vi "ResonanceAnalyzer.vi"() -> ()   [LabVIEW 2014]
uses:
  <vilib>/imath/engines/lvmath2/RunTimeEngine/Managers/WorkSpace/UID Generator.vi
  <vilib>/imath/engines/lvmath2/RunTimeEngine/RangeToken/NIMS_Range.vi
  <instcachedir>/0/NIMS_Range_9BCE657718DF4976A877346C61F22738.lvgen/NIMS_Range_9BCE657718DF4976A877346C61F22738_000.vi
  <vilib>/imath/engines/lvmath2/RunTimeEngine/RunTimeType/NIMS_RunTimeType_From StrictType (excl LVString).vi
  <instcachedir>/0/NIMS_RunTimeType_From StrictType (excl LVString)_15A5391EEA9C4AACB9955AC755B83D29.lvgen/NIMS_RunTimeType_From StrictType (excl LVString)_15A5391EEA9C4AACB9955AC755B83D29_000.vi
  <vilib>/imathl/engines/lvmath/Functions/Error Handling/Create Error.vi
  <vilib>/imath/engines/lvmath2/RunTimeEngine/LocalVariableDefStatement/MC_LocalVariableDefStatement_Display.vi
  <vilib>/imath/engines/lvmath2/RunTimeEngine/ArithmeticOperatorToken/NIMS_ArithmeticOperator_minus.vi
  <instcachedir>/0/NIMS_ArithmeticOperator_minus_39C0593E74DA4138ACA2AB742906488D.lvgen/NIMS_ArithmeticOperator_minus_39C0593E74DA4138ACA2AB742906488D_003.vi
  <vilib>/imath/engines/lvmath2/RunTimeEngine/BuiltInFunctions/randnormal/NIMS_randnormal(1,I32).vi
  <vilib>/imath/engines/lvmath2/RunTimeEngine/ErrorHandling/NIMS_Error From Error Code.vi
  <vilib>/imath/engines/lvmath2/RunTimeEngine/ArithmeticOperatorToken/NIMS_ArithmeticOperator_power(S).vi
  <instcachedir>/0/NIMS_ArithmeticOperator_power(S)_CAFE680B12A64A3A8F5E28A20C679B7D.lvgen/NIMS_ArithmeticOperator_power(S)_CAFE680B12A64A3A8F5E28A20C679B7D_014.vi
  <vilib>/imath/engines/lvmath2/RunTimeEngine/ArithmeticOperatorToken/NIMS_ArithmeticOperator_plus.vi
  <instcachedir>/0/NIMS_ArithmeticOperator_plus_48D6EAACA5D645B09F7EC9C016C2DEA8.lvgen/NIMS_ArithmeticOperator_plus_48D6EAACA5D645B09F7EC9C016C2DEA8_000.vi
  <vilib>/imath/engines/lvmath2/RunTimeEngine/ErrorHandling/NIMS_Create Error From Enums.vi
  <vilib>/imath/engines/lvmath2/RunTimeEngine/Managers/SymbolTable/Clear UID.vi
  <vilib>/imath/engines/lvmath2/RunTimeEngine/NodeEndStatement/NIMS_NodeEndStatement_Output.vi
  <instcachedir>/0/NIMS_NodeEndStatement_Output_53EC0D466D134D7ABD903AC30B43404B.lvgen/NIMS_NodeEndStatement_Output_53EC0D466D134D7ABD903AC30B43404B_000.vi
  <instcachedir>/0/NIMS_NodeEndStatement_Output_53EC0D466D134D7ABD903AC30B43404B.lvgen/NIMS_NodeEndStatement_Output_53EC0D466D134D7ABD903AC30B43404B_005.vi
  <vilib>/imath/engines/lvmath2/RunTimeEngine/ErrorHandling/NIMS_Finalize Error.vi
  <vilib>/Utility/file.llb/Read From Spreadsheet File (DBL).vi
  <vilib>/imath/engines/lvmath2/RunTimeEngine/Managers/SymbolTable/NIMS_WorkSpace.lvlib
panel:
  out "output cluster":cluster{"all rows":dbl[], "Array":dbl[]}={"all rows"=[425.0, 430.0, 435.0, 440.0, 445.0, 450.0, 455.0, 460.0, 465.0, 470.0, 475.0, 480.0, 485.0, 490.0, 495.0, 500.0, 505.0, 510.0, 515.0, 520.0, 525.0, 530.0, 535.0, 540.0, 545.0, 550.0, 555.0, 560.0, 565.0], "Array"=[0.00029010896046823345, 0.000307774576785936, 0.00032832543217633636, 0.0003525272075386067, 0.0003814382755160812, 0.000416561323783634, 0.0004600972655461633, 0.0005153884048945562, 0.0005877272439052437, 0.0006858979557065526, 0.0008251875476773748, 0.0010328740074356068, 0.0013523841688152917, 0.0017892153610694526, 0.0020107857493675313, 0.0016828151148900047, 0.0012753396459793623, 0.0009947134075484914, 0.0008111662113022912, 0.0006861595529584501, 0.0005967970519750586, 0.0005301782426142894, 0.0004787804413681282, 0.00043800311684869474, 0.0004049022123545997, 0.00037751685257886314, 0.00035449514124371066, 0.000334876933310768, 0.0003179625943458466]}
  out "XY Graph":cluster{dbl[], dbl[]}[](graph)=[{[425.0, 430.0, 435.0, 440.0, 445.0, 450.0, 455.0, 460.0, 465.0, 470.0, 475.0, 480.0, 485.0, 490.0, 495.0, 500.0, 505.0, 510.0, 515.0, 520.0, 525.0, 530.0, 535.0, 540.0, 545.0, 550.0, 555.0, 560.0, 565.0], [0.00032, 0.00034, 0.00034, 0.00036, 0.0004, 0.0004, 0.00046, 0.0005, 0.00059, 0.00066, 0.00082, 0.00102, 0.00141, 0.00177, 0.00199, 0.00173, 0.00124, 0.00103, 0.00079, 0.00067, 0.00061, 0.00051, 0.00046, 0.00039, 0.00041, 0.00036, 0.00037, 0.00035, 0.00032]}, {[425.0, 430.0, 435.0, 440.0, 445.0, 450.0, 455.0, 460.0, 465.0, 470.0, 475.0, 480.0, 485.0, 490.0, 495.0, 500.0, 505.0, 510.0, 515.0, 520.0, 525.0, 530.0, 535.0, 540.0, 545.0, 550.0, 555.0, 560.0, 565.0], [0.00029010896046823345, 0.000307774576785936, 0.00032832543217633636, 0.0003525272075386067, 0.0003814382755160812, 0.000416561323783634, 0.0004600972655461633, 0.0005153884048945562, 0.0005877272439052437, 0.0006858979557065526, 0.0008251875476773748, 0.0010328740074356068, 0.0013523841688152917, 0.0017892153610694526, 0.0020107857493675313, 0.0016828151148900047, 0.0012753396459793623, 0.0009947134075484914, 0.0008111662113022912, 0.0006861595529584501, 0.0005967970519750586, 0.0005301782426142894, 0.0004787804413681282, 0.00043800311684869474, 0.0004049022123545997, 0.00037751685257886314, 0.00035449514124371066, 0.000334876933310768, 0.0003179625943458466]}]
  out "Results":T1={"Amplitude"=0.001938254361984839, "Q"=7.806460499651551e-05, "Center Frequency"=494.37424166547555}
  in  "?":enum32{"Simulation", "Experiment"}(tab)=enum."Experiment"
  in  "Input Parameters":T2={"Q"=10.0, "Center Frequency"=600.0, "Start Frequency"=400.0, "End Frequency"=800.0, "df"=5.0, "Noise Level"=0.01}
  in  "file path (dialog if empty)":path=path "C:/Users/eclifton/Documents/GitHub/week7/Impulse Data2.txt"
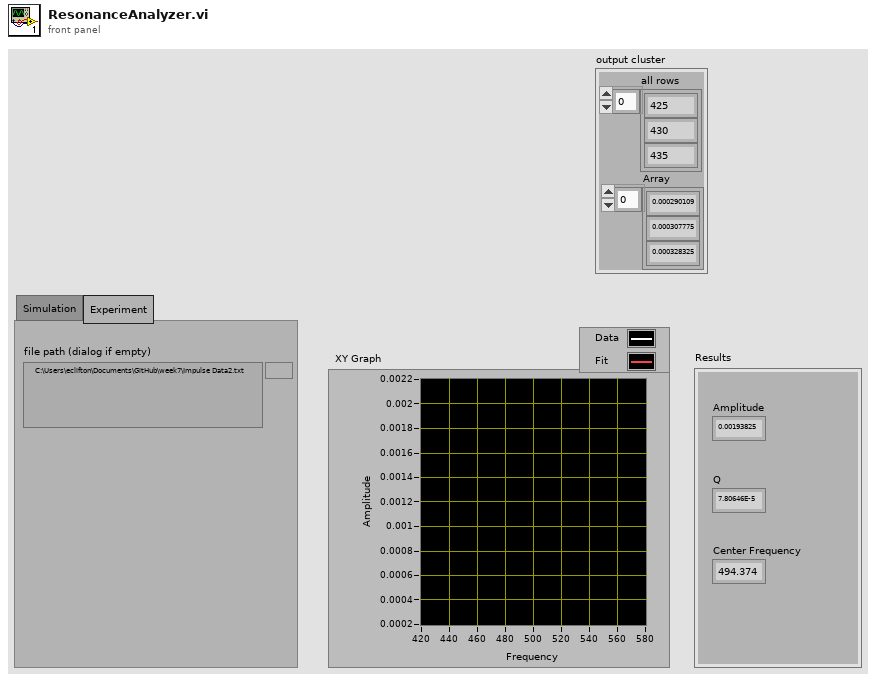
[diagram p1: front panel]
types:
  T1 = cluster{"Amplitude":dbl, "Q":dbl, "Center Frequency":dbl}
  T2 = cluster{"Q":dbl, "Center Frequency":dbl, "Start Frequency":dbl, "End Frequency":dbl, "df":dbl, "Noise Level":dbl}
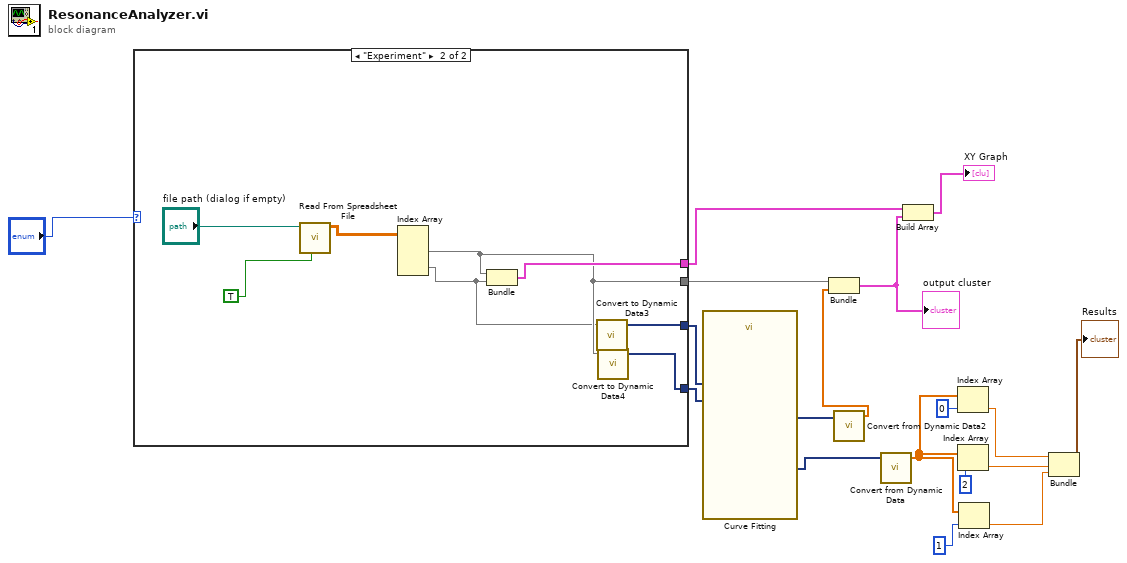
[diagram p0: block diagram]
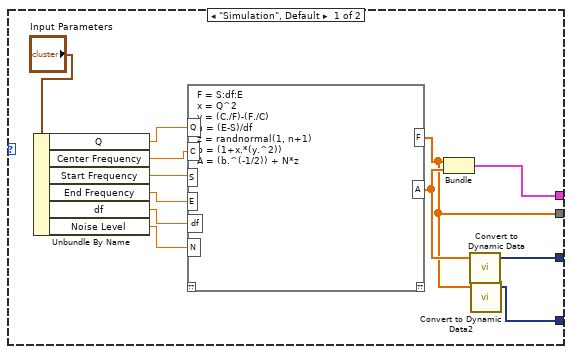
[diagram p2: hidden frame]
diagram:
  n1 = case shown="\"Experiment\"" "?" {
    tunnel: [w23 w237] -> w6
    tunnel: [w21 w235] -> w17
    tunnel: [w20 w234] -> w16
    tunnel: [w19 w233] -> w2
    frame "Simulation", Default {
      n2 = Unbundle By Name("Input Parameters") -> ("Q"=w25:dbl, "Center Frequency"=w24:dbl, "Start Frequency"=w29:dbl, "End Frequency"=w28:dbl, "df"=w27:dbl, "Noise Level"=w26:dbl)
      n3 = mathscript code="F = S:df:E\nx = Q^2\ny = (C./F)-(F./C)\nn = (E-S)/df\nz = randnormal(1, n+1)\nb = (1+x.*(y.^2))\nA = (b.^(-1/2)) + N*z"("S"=w29, "Q"=w25, "C"=w24, "E"=w28, "df"=w27, "N"=w26) -> ("F"=w19:dbl[], "A"=w22:cdb[])  [unwired: 1 in, 1 out]
      n4 = Bundle("F"=w19, "A"=w22) -> (w23:cluster{"F":dbl[], "A":cdb[]})  [unwired: 1 in]
      n5 = call "Convert to Dynamic Data"("Array"=w22) -> ("Dynamic Data Type"=w21:dynamicdata)  [unwired: 3 in]
      n6 = call "Convert to Dynamic Data2"("Array"=w19) -> ("Dynamic Data Type"=w20:dynamicdata)  [unwired: 3 in]
    }
    frame "Experiment" {
      n7 = call-poly <vilib>:"Read From Spreadsheet File.vi"("transpose (no:F)"=TRUE, "file path (dialog if empty)"="file path (dialog if empty)") -> ("all rows"=w239:dbl[][])  [unwired: 5 in, 4 out]
      n8 = Index Array(array=w239) -> (element #1=w233:dbl[], element #2=w232:dbl[])  [unwired: 4 in]
      n9 = Bundle("all rows"=w233, "all rows"=w232) -> (w237:cluster{"all rows":dbl[], "all rows":dbl[]})  [unwired: 1 in]
      n10 = call "Convert to Dynamic Data3"("Array"=w232) -> ("Dynamic Data Type"=w235:dynamicdata)  [unwired: 3 in]
      n11 = call "Convert to Dynamic Data4"("Array"=w233) -> ("Dynamic Data Type"=w234:dynamicdata)  [unwired: 3 in]
    }
  }
  n12 = call "Curve Fitting"("Locations"=w16, "Signals"=w17) -> ("best fit"=w4:dynamicdata, "non-linear coefficients"=w15:dynamicdata)  [unwired: 5 in, 3 out]
  n13 = call "Convert from Dynamic Data2"("Dynamic Data Type"=w4) -> ("Array"=w3:dbl[])  [unwired: 3 in]
  n14 = Bundle("all rows"=w2, "Array"=w3) -> (w1:cluster{"all rows":dbl[], "Array":dbl[]})  [unwired: 1 in]
  "output cluster" <- w1
  n15 = call "Convert from Dynamic Data"("Dynamic Data Type"=w15) -> ("Array"=w12:dbl[])  [unwired: 3 in]
  n16 = Build Array(w6, w1) -> (→"XY Graph":cluster{"all rows":dbl[], "A":cdb[]}[])
  n17 = Index Array(array=w12, index=0) -> (element=w10:dbl)
  n18 = Index Array(array=w12, index=2) -> (element=w9:dbl)
  n19 = Index Array(array=w12, index=1) -> (element=w8:dbl)
  n20 = Bundle(w10, w9, w8) -> (→"Results":cluster{dbl, dbl, dbl})  [unwired: 1 in]
